vi "Global_SEN_Data Out.vi"() -> ()   [LabVIEW 2023, in "NTV Read Write.lvlib"]
uses:
  NTV Read Write.lvlib
panel:
  in  "SEN_Template_BoolDataIn":bool
  in  "SEN_Template_CycleTime(S)":dbl
  in  "SEN_Template_DBLDataOut":dbl
  # "The Names of the Data items in the Global Variable MUST describe who the Single Writer is\nFor Sensor Globals the the naming convention is\n   \nSEN_Lib Name_Data Name\n\nExamples:\nSEN_Gyro_Angle\nSEN_Sonar_Distance"
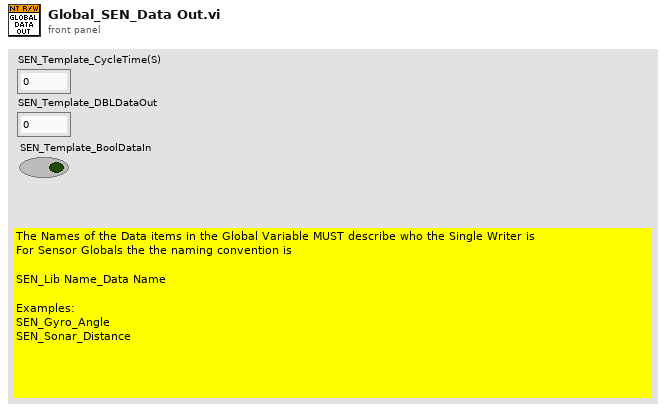
[diagram p1: front panel]
diagram:
